vi "8-bit video export-Get cursors location.vi"() -> (1 "Cursors location":T1)   [LabVIEW 2017]
uses:
  Globals/gl_Time series viewer globals.vi
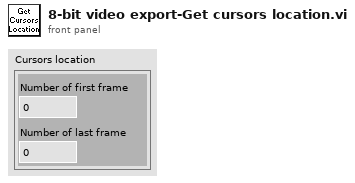
[diagram p1: front panel]
types:
  T1 = cluster{"Number of first frame":i32, "Number of last frame":i32}
  T2 = typedef "Time series viewer refs.ctl" = cluster{"This VI":refnum<vi>, "Image control":refnum<vi>, "AVI Mode ind":refnum<vi>, "Play":refnum<vi>, "Stop":refnum<vi>, "Back":refnum<vi>, "Scrollbar":refnum<vi>, "Video length info":refnum<vi>, "Expected speed values":refnum<vi>, "Intensity":refnum<vi>, "Path":refnum<vi>, "Selection sliders":refnum<vi>, "Speed Graph ref":refnum<vi>, "Frame rate set (fps)":refnum<vi>, "Channel to load":refnum<vi>, "Number of rows to generate":refnum<vi>, "Colour":refnum<vi>}
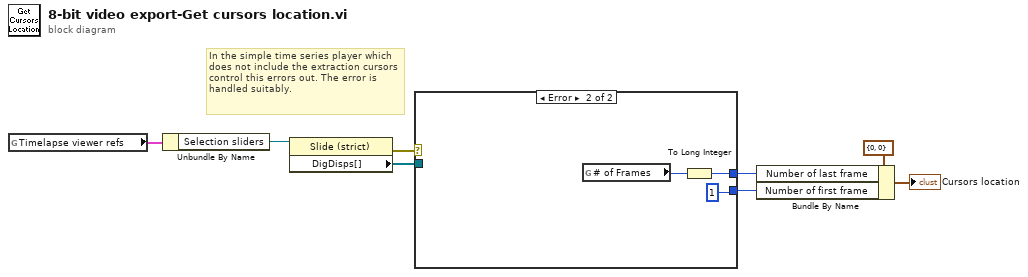
[diagram p0: block diagram]
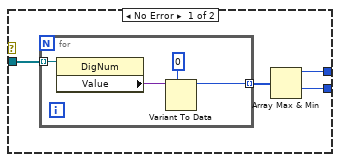
[diagram p2: hidden frame]
diagram:
  # "In the simple time series player which does not include the extraction cursors control this errors out. The error is handled suitably."
  n1 = global read "gl_Time series viewer globals.vi" "Timelapse viewer refs"() -> (w3:T2)
  n2 = Unbundle By Name(w3) -> ("Selection sliders"=w2:refnum<vi>)
  n3 = property on="Property Node" class="Slide (strict)"(reference=w2) -> (error out=w1:errorcluster, "DigDisps[]"=w8:refnum<vi>[])  [unwired: 1 in, 1 out]
  n4 = case shown="Error" w1 {
    tunnel: w8 -> [w12 _]
    tunnel: [w10 1] -> w6
    tunnel: [w9 w17] -> w4
    frame No Error {
      n5 = for {
        tunnel: w12 -> [w16] mode=indexing
        tunnel: [w13] -> w11 mode=indexing
        n6 = property class="DigNum"(reference=w16) -> ("Value"=w15:variant)  [unwired: 1 in, 2 out]
        n7 = Variant To Data(type=0 ("Value"), Variant=w15) -> (data=w13:i32)  [unwired: 1 in, 1 out]
      }
      n8 = Array Max & Min(array=w11) -> (max value=w9:i32, min value=w10:i32)  [unwired: 2 out]
    }
    frame Error {
      n9 = global read "gl_Time series viewer globals.vi" "# of Frames"() -> (w19:u32)
      n10 = To Long Integer(number=w19) -> (32bit integer=w17:i32)
    }
  }
  n11 = Bundle By Name(cluster=T1 {"Number of first frame"=0, "Number of last frame"=0} ("Cluster"), "Number of last frame"=w4, "Number of first frame"=w6) -> (→"Cursors location":T1)
